vi "Remove Object By ID.vi"(8 "error in (no error)":errorcluster, 10 "ID":i32=-1, 11 "Objects in":refnum<class "Objects.lvclass">) -> (0 "error out":errorcluster, 3 "Objects out":refnum<class "Objects.lvclass">)   [LabVIEW 2019, in "HierDAL Library.lvlib" / "Database.lvlib" / "Repositories.lvlib" / "Objects.lvclass"]
uses:
  Objects.lvclass
  Objects.lvclass/Objects.ctl
  Database Manager Class/Database Manager.lvclass
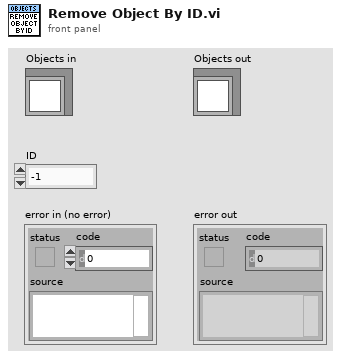
[diagram p1: front panel]
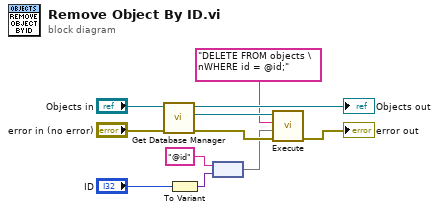
[diagram p0: block diagram]
diagram:
  n1 = call "Get Database Manager.vi"("error in (no error)"="error in (no error)", "Objects in"="Objects in") -> ("error out"=w8:errorcluster, "Database Manager"=w7:refnum<class "Database Manager.lvclass">, "Objects out"=→"Objects out":refnum<class "Objects.lvclass">)  [unwired: 7 in]
  n2 = To Variant(anything="ID") -> (Variant=w4:variant)
  n3 = node("@id" ("key"), w4) -> (w5:map{string, variant})
  n4 = call-dynamic "Execute.vi"("error in (no error)"=w8, "Parameters"=w5, "Query"="DELETE FROM objects \nWHERE id = @id;", "Database Manager in"=w7) -> ("error out"=→"error out":errorcluster)  [unwired: 5 in, 2 out]
